vi "height_flight.vi"(1 "t":dbl) -> (0 "h":dbl)   [LabVIEW 2013]
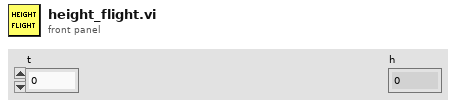
[diagram p1: front panel]
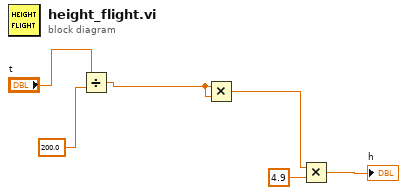
[diagram p0: block diagram]
diagram:
  n1 = Divide(x="t", y=200.0) -> (x/y=w4:dbl)
  n2 = Multiply(x=w4, y=w4) -> (x*y=w3:dbl)
  n3 = Multiply(x=w3, y=4.9) -> (x*y=→"h":dbl)
